vi "Untitled 2.vi"() -> ()   [LabVIEW 2020]
uses:
  <vilib>/Utility/file.llb/Read Delimited Spreadsheet (string).vi
  <vilib>/Utility/file.llb/Write Delimited Spreadsheet (string).vi
  28b294ec-0788-41a7-96e6-a65b3b29f992.vi
panel:
  in  "file path (dialog if empty)":path
  in  "Enable":bool
  out "error out":errorcluster
  out "Cluster Out":T1
  out "VISA out":refnum<visa-resource-name>
  in  "error in":errorcluster
  in  "Cluster":T1
  in  "VISA Refnum in":refnum<visa-resource-name>
  out "Array 2":string[](array[string])
  out "Array":T2(array[cluster])
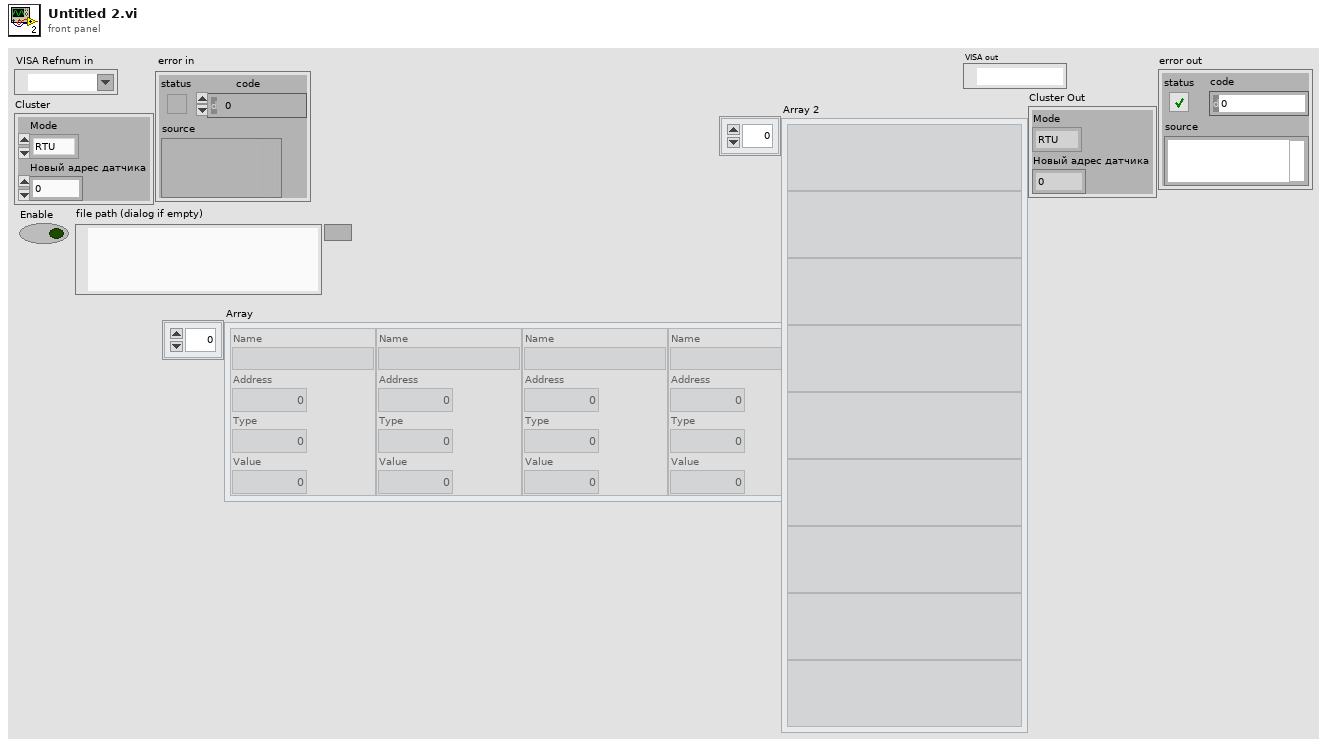
[diagram p1: front panel]
types:
  T1 = cluster{"Mode":enum16{"RTU", "ASCII"}, "Новый адрес датчика":u16}
  T2 = cluster{"Name":string, "Address":u16, "Type":u16, "Value":sgl}[]
  T3 = cluster{"Name":string, "Address":u16, "Type":u16, "Value":sgl}
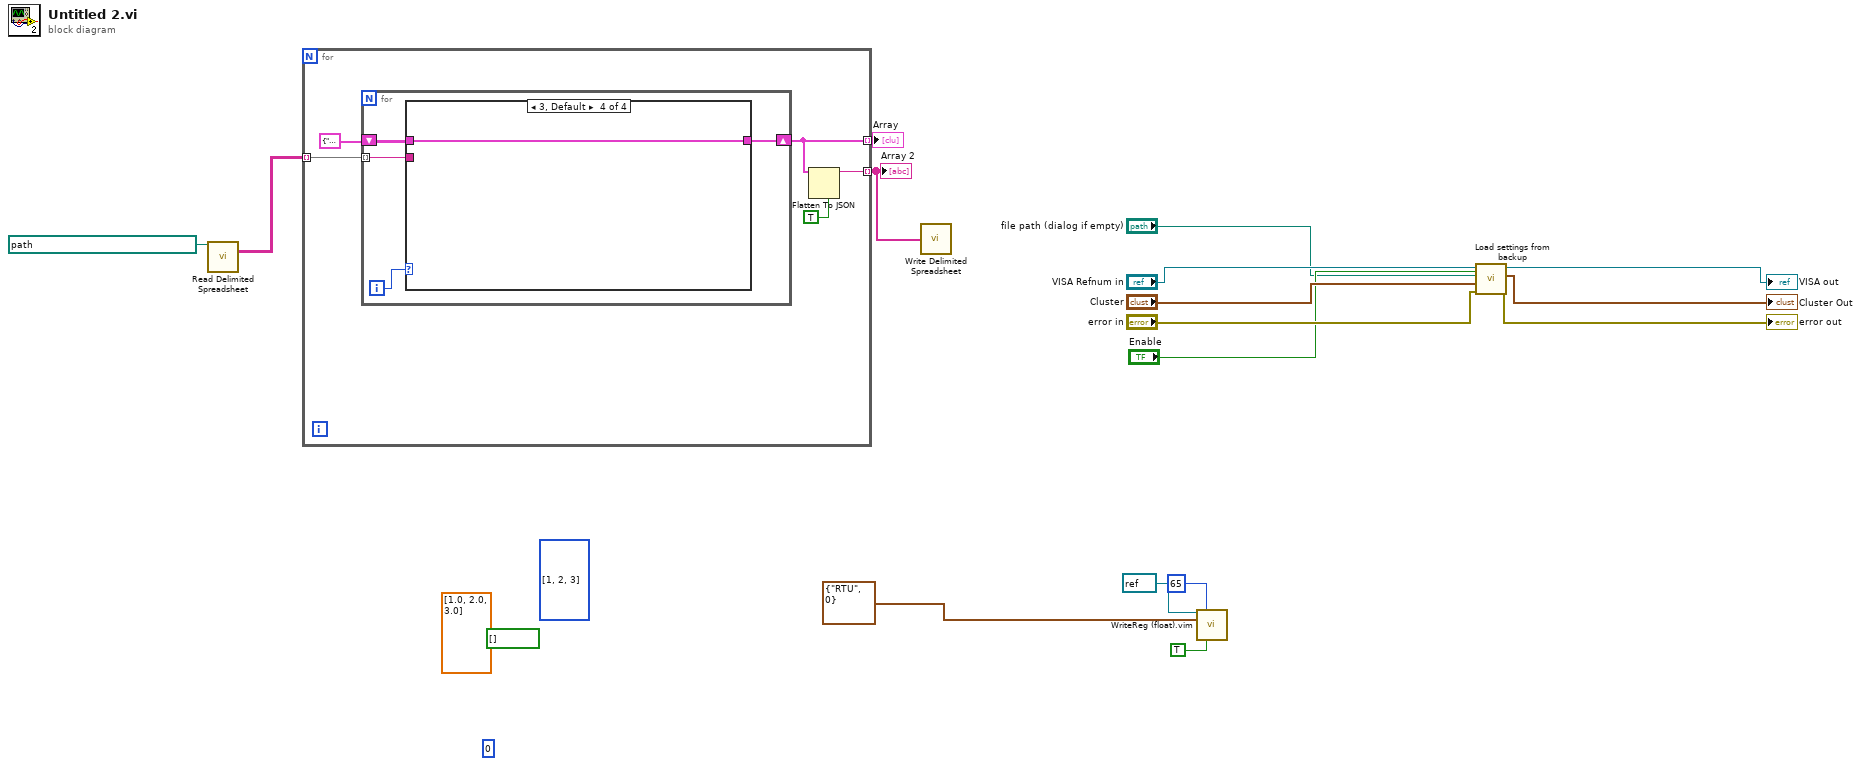
[diagram p0: block diagram]
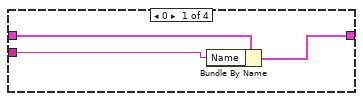
[diagram p2: hidden frame]
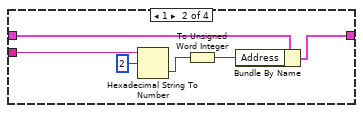
[diagram p3: hidden frame]
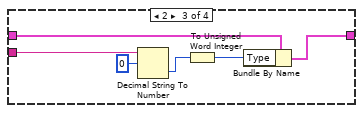
[diagram p4: hidden frame]
diagram:
  (unwired) bool[] []
  (unwired) u16[] [1, 2, 3]
  (unwired) u16 0
  (unwired) sgl[] [1.0, 2.0, 3.0]
  n1 = call-poly <vilib>:"Read Delimited Spreadsheet.vi"("file path (dialog if empty)"=path "E:/lv projects/toolbox/Книга1.txt") -> ("all rows"=w16:string[][])  [unwired: 9 in, 5 out]
  n2 = for {
    tunnel: w16 -> [w21] mode=indexing
    tunnel: [w19] -> w10 mode=indexing
    tunnel: [w18] -> w9 mode=indexing
    n3 = for {
      tunnel: w21 -> [w22] mode=indexing
      shift-right: [w23] -> w19
      shift-left: T3 {"Name"="", "Address"=0, "Type"=0, "Value"=0.0} -> [w25]
      i -> [w24]
      n4 = case shown="3, Default" w24 {
        tunnel: w25 -> [w28 w34 w40 w41]
        tunnel: [w27 w33 w39 w41] -> w23
        tunnel: w22 -> [w26 w32 w38 _]
        frame 0 {
          n5 = Bundle By Name(cluster=w28, "Name"=w26) -> (w27:T3)
        }
        frame 1 {
          n6 = Hexadecimal String To Number(string=w32, offset=2) -> (number=w30:u32)  [unwired: 1 in, 1 out]
          n7 = To Unsigned Word Integer(number=w30) -> (unsigned 16bit integer=w29:u16)
          n8 = Bundle By Name(cluster=w34, "Address"=w29) -> (w33:T3)
        }
        frame 2 {
          n9 = Decimal String To Number(string=w38, offset=0) -> (number=w36:i32)  [unwired: 1 in, 1 out]
          n10 = To Unsigned Word Integer(number=w36) -> (unsigned 16bit integer=w35:u16)
          n11 = Bundle By Name(cluster=w40, "Type"=w35) -> (w39:T3)
        }
        frame 3, Default {
        }
      }
    }
    n12 = Flatten To JSON(enable LabVIEW extensions? (T)=TRUE, anything=w19) -> (JSON string=w18:string)  [unwired: 1 in, 1 out]
  }
  "Array" <- w10
  "Array 2" <- w9
  n13 = call-poly <vilib>:"Write Delimited Spreadsheet.vi"("1D data"=w9) -> ()  [unwired: 13 in, 2 out]
  n14 = call "WriteReg (float).vim"("VISA Refnum in"=refnum<visa-resource-name> refnum, "Address"=u16 65, "Cluster"=T1 {"Mode"=enum."RTU", "Новый адрес датчика"=0}, "Enable"=TRUE) -> ()  [unwired: 9 in, 3 out]
  n15 = call "Load settings from backup.vi"(7:"Enable", "error in (no error)"="error in", "file path (dialog if empty)"="Cluster", "Cluster in"="file path (dialog if empty)", "VISA Refnum in"="VISA Refnum in") -> ("error out"=→"error out":errorcluster, "Cluster out"=→"Cluster Out":T1, "VISA Refnum out"=→"VISA out":refnum<visa-resource-name>)  [unwired: 4 in]
